vi "5650+SR830+1022.vi"() -> ()   [LabVIEW 2019]
uses:
  lib/Stanford Research 830/Public/Data/Read (All Parameters).vi
  <vilib>/Utility/file.llb/Write Delimited Spreadsheet (string).vi
  lib/Stanford Research 830/Stanford Research 830.lvlib
  SubVI/SubVI.lvlib
panel:
  out "output array":string[](array[string])
  out "Read Buffer":string
  in  "Timeout":u32=1000
  out "Serial Versions":string
  in  "file path (use dialog)":path
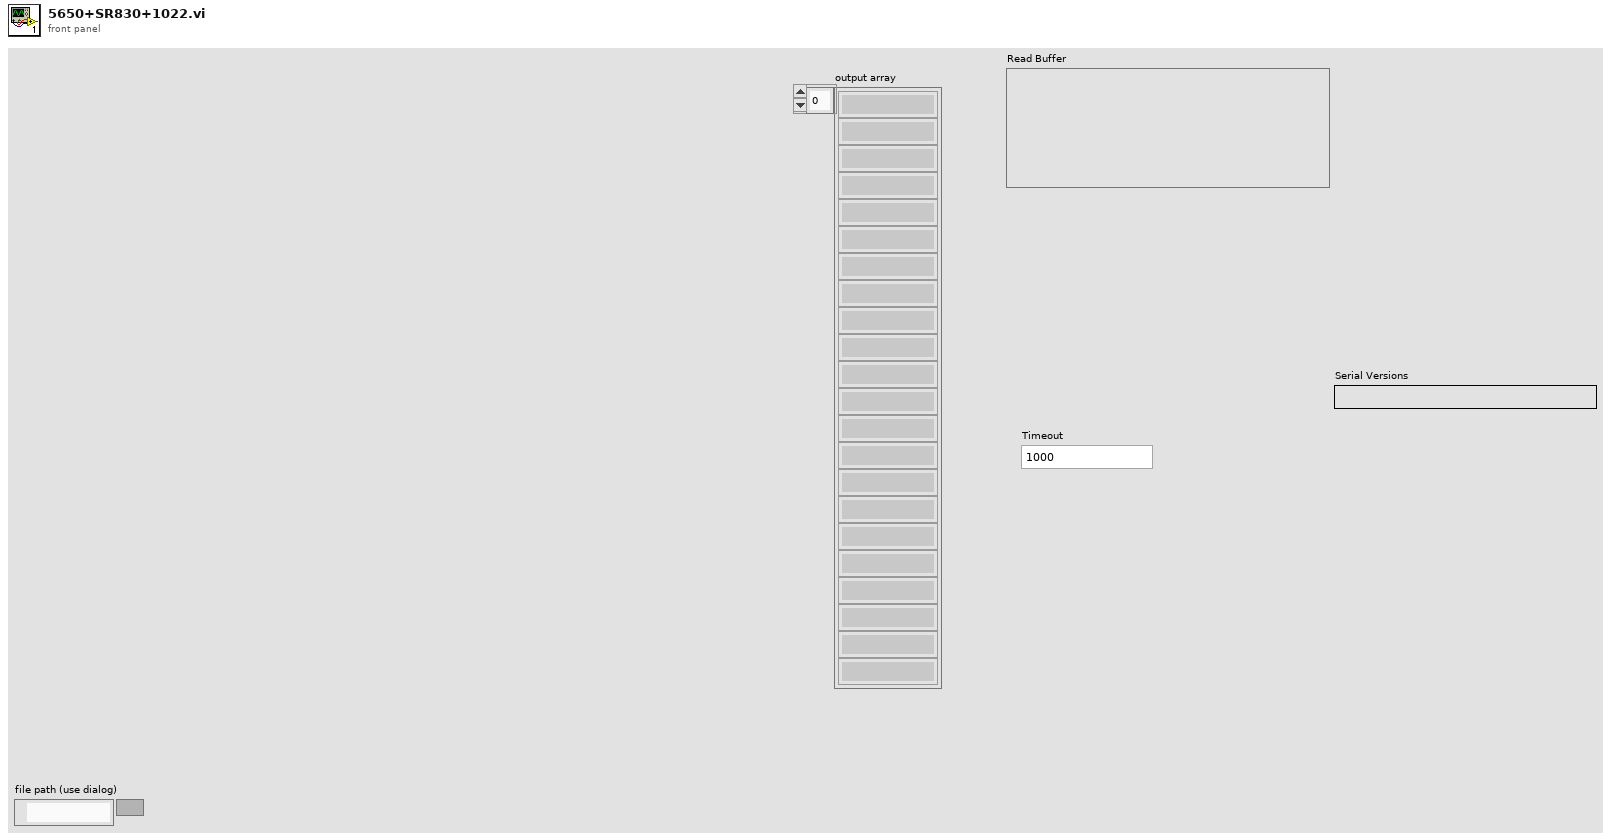
[diagram p1: front panel]
types:
  T1 = enum16{"open", "replace", "create", "open or create", "replace or create", "replace or create with confirmation"}
  T2 = cluster{"X-Value":dbl, "Y-Value":dbl, "R-Value":dbl, "Theta-Value":dbl, "Aux In 1 Value":dbl, "Aux In 2 Value":dbl, "Aux In 3 Value":dbl, "Aux In 4 Value":dbl, "Reference Frequency":dbl, "Channel 1 Display":dbl, "Channel 2 Display":dbl}
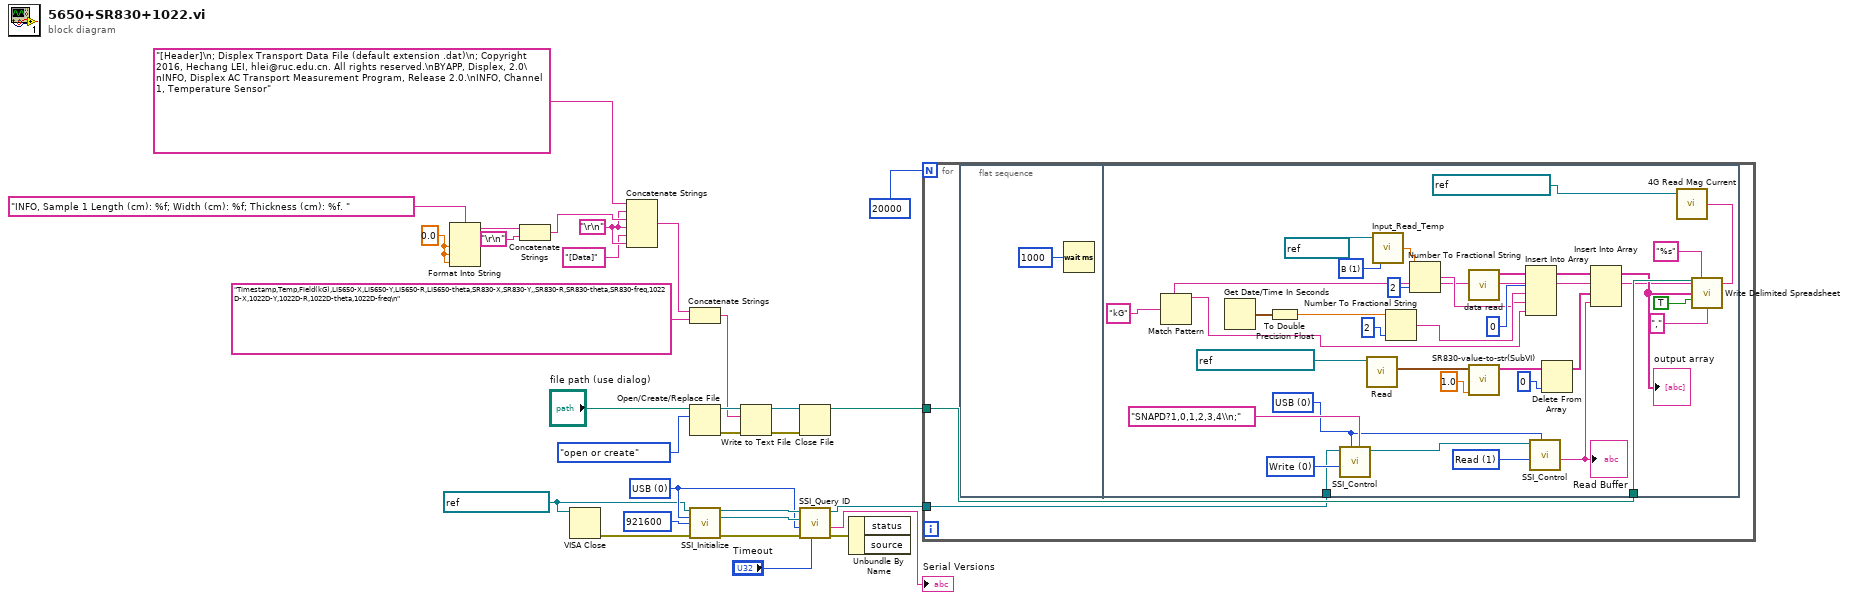
[diagram p0: block diagram]
diagram:
  w6 = u16 0 items=["USB", "RS232", "GPIB"] ("Remote Mode")
  w3 = refnum<visa-resource-name> "ASRL7::INSTR" ("VISA resource name")
  w19 = 0.0 ("输入 1")
  w22 = "\r\n"
  n1 = Format Into String(format string="INFO, Sample 1 Length (cm): %f; Width (cm): %f; Thickness (cm): %f. " ("string"), w19, w19, w19) -> (resulting string=w26:string)  [unwired: 2 in, 1 out]
  n2 = Concatenate Strings(w26, "\r\n") -> (w27:string)
  n3 = VISA Close(VISA resource name=w3) -> (error out=w2:errorcluster)  [unwired: 1 in]
  n4 = Concatenate Strings("[Header]\n; Displex Transport Data File (default extension .dat)\n; Copyright 2016, Hechang LEI, hlei@ruc.edu.cn. All rights reserved.\nBYAPP, Displex, 2.0\nINFO, Displex AC Transport Measurement Program, Release 2.0.\nINFO, Channel 1, Temperature Sensor" ("string"), w22, w27, w22, "[Data]" ("string"), w22) -> (w28:string)
  n5 = Concatenate Strings(w28, "Timestamp,Temp,Field(kG),LI5650-X,LI5650-Y,LI5650-R,LI5650-theta,SR830-X,SR830-Y,,SR830-R,SR830-theta,SR830-freq,1022D-X,1022D-Y,1022D-R,1022D-theta,1022D-freq\n" ("字符串")) -> (w18:string)
  n6 = Open/Create/Replace File(file path (use dialog)="file path (use dialog)", operation (0:open)=T1."open or create") -> (refnum out=w29:refnum<file>, error out=w15:errorcluster)  [unwired: 4 in, 1 out]
  n7 = call "SSI_Initialize.vi"("VISA resource name"=w3, "Remote Mode"=w6, "baud rate (921600)"=u32 921600 ("Baud rate (921600)"), "error in (no error)"=w2) -> ("VISA resource name out"=w10:refnum<visa-resource-name>, "connection ID(Ethernet)"=w9:refnum<k5>, "error out"=w8:errorcluster)  [unwired: 9 in]
  n8 = Write to Text File(file (use dialog)=w29, text=w18, error in=w15) -> (refnum out=w17:refnum<file>, error out=w16:errorcluster)  [unwired: 1 in, 1 out]
  n9 = Close File(refnum=w17, error in=w16) -> (path=w14:path)  [unwired: 1 out]
  n10 = call "SSI_Query ID.vi"("Timeout"="Timeout", "Error in (no error)"=w8, "Remote Mode"=w6, "Connection ID in"=w9, "VISA resource name"=w10) -> ("Error out"=w5:errorcluster, "Read Buffer"=→"Serial Versions":string, "VISA resource  out"=w1:refnum<visa-resource-name>)  [unwired: 3 in, 1 out]
  n11 = Unbundle By Name(w5) -> ()  [unwired: 2 out]
  n12 = for {
    N: 20000 -> [_]
    tunnel: w14 -> [w32]
    tunnel: w1 -> [w31]
    n13 = flat-sequence {
      tunnel: w32 -> [w67]
      tunnel: w31 -> [w56]
      frame #0 {
        n14 = Wait (ms)(milliseconds to wait=u32 1000) -> ()  [unwired: 1 out]
      }
      frame #1 {
        w41 = u8 1 items=["A", "B", "C", "D"] ("Input")
        w55 = u16 1 items=["Write", "Read"] ("Control")
        w57 = u16 0 items=["Write", "Read"] ("Control")
        w58 = u16 0 items=["USB", "RS232", "GPIB", "Ethernet"] ("Remote Mode")
        n15 = Get Date/Time In Seconds() -> (seconds since 1Jan1904=w51:timestamp)
        n16 = To Double Precision Float(number=w51) -> (double precision float=w50:dbl)
        n17 = call "SSI_Control.vi"("Write Buffer"="SNAPD?1,0,1,2,3,4\\n;", "Remote Mode"=w58, "Control"=w57, "VISA resource name"=w56) -> ("VISA resource  out"=w60:refnum<visa-resource-name>)  [unwired: 4 in, 3 out]
        n18 = call-poly "Read.vi"("VISA resource name"=refnum<visa-resource-name> "GPIB1::1::INSTR") -> ("Parameter Values"=w62:T2)  [unwired: 8 in, 2 out]
        n19 = call "Input_Read_Temp.vi"("Input"=w41, "VISA In"=refnum<visa-resource-name> "COM3") -> ("Temperature"=w40:dbl)  [unwired: 1 in, 2 out]
        n20 = Number To Fractional String(number=w50, precision (6)=i16 2) -> (F-format string=w44:string)  [unwired: 2 in]
        n21 = Number To Fractional String(number=w40, precision (6)=i16 2) -> (F-format string=w38:string)  [unwired: 2 in]
        n22 = call "data read.vi"() -> ("F-format string"=w46:string[])  [unwired: 11 in]
        n23 = call "SR830-value-to-str(SubVI).vi"("电流"=1.0, "Parameter Values"=w62) -> ("数组"=w48:string[])  [unwired: 9 in]
        n24 = call "SSI_Control.vi"("Remote Mode"=w58, "Control"=w55, "VISA resource name"=w60) -> ("Read Buffer"=w54:string)  [unwired: 5 in, 3 out]
        "Read Buffer" <- w54
        n25 = Delete From Array(array=w48, index=0) -> (array with subset deleted=w52:string[])  [unwired: 1 in, 1 out]
        n26 = call "4G Read Mag Current.vi"("VISA session"=refnum<visa-resource-name> "GPIB0::1::INSTR") -> ("response out"=w37:string)  [unwired: 2 in, 2 out]
        n27 = Match Pattern(string=w37, regular expression="kG" ("正则表达式")) -> (before substring=w34:string)  [unwired: 1 in, 3 out]
        n28 = Insert Into Array(array=w46, index=0, new element #1=w44, new element #2=w38, new element #3=w34) -> (w43:string[])
        n29 = Insert Into Array(array=w43, new element #1=w52, new element #2=w54) -> (w63:string[])  [unwired: 1 in]
        "output array" <- w63
        n30 = call-poly <vilib>:"Write Delimited Spreadsheet.vi"("file path (dialog if empty)"=w67, "format (%s)"="%s" ("format (%.3f)"), "1D data"=w63, "append to file? (new file:F)"=TRUE, "delimiter (\\t)"="," ("delimiter (\\t)")) -> ()  [unwired: 9 in, 2 out]
      }
    }
  }
